vi "Request UI Display--template.vi"(6 "wait for reply (T)":bool=TRUE, 8 "error in (no error)":errorcluster, 10 "Scenario":T1) -> (0 "error out":errorcluster, 3 "Accept?":bool)   [LabVIEW 2014, in "hse-dqmh-dynamicrequesters.lvlib"]
uses:
  hse-dqmh-dynamicrequesters.lvlib
  Controls/Module Display Scenarios.ctl
  hse-dqmh.lvlib
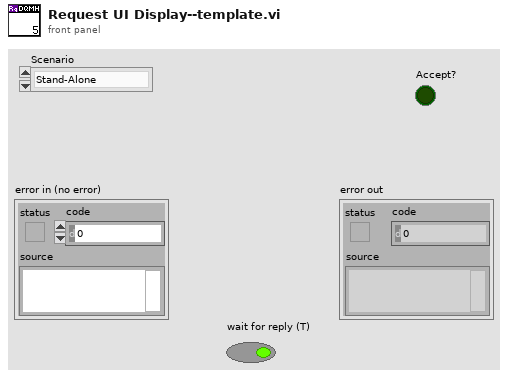
[diagram p1: front panel]
types:
  T1 = typedef "hse-dqmh.lvlib/Module Display Scenarios.ctl" = enum16{"Stand-Alone", "Managed"}
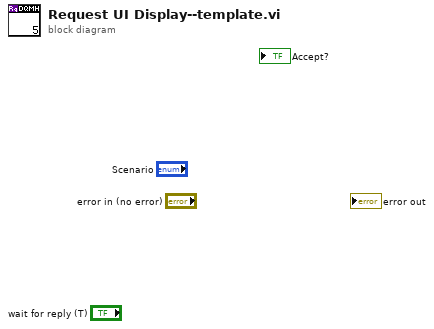
[diagram p0: block diagram]
diagram:
